vi "Test.vi"() -> ()   [LabVIEW 2014]
doc: "This VI is called when test mode begins, and will automatically be terminated when it ends. You can add manual or automatic tests and invoke them from the dashboard."
uses:
  Robot Global Data.vi
  <vilib>/Rock Robotics/WPI/MotorControl/WPI_MotorControlOpenCANTalonSRX.vi
  <vilib>/Rock Robotics/Network Tables/SD Read String Array.vi
panel:
  in  "Stop":bool
  in  "Motor Power":dbl format="%#_13g"
  in  "Motor":i32(listbox)
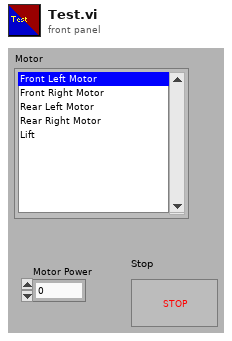
[diagram p1: front panel]
types:
  T1 = typedef "WPI_MotorControlDeviceRef.ctl" = cluster{"DeviceStatus":errorcluster, "Type":T2, "PWM":cluster{"Controller":T3, "PWM Channel":T4, "DeadBand":T5}, "CAN":cluster{"Device Number":u8, "Control Mode":T6, "Semaphore":T7, "Max Vout":dbl, "TalonSRX Control Mode":T8}, "Invert":bool, "TransformRef":T9, "InvTransformRef":T9}
  T2 = typedef "WPI_MotorControlType.ctl" = enum16{"PWM", "CAN", "CANTalonSRX"}
  T3 = typedef "FPGA_TypedefDigitalModule.ctl" = enum16{"Controller 1"}
  T4 = typedef "FPGA_DIOPWMChannel.ctl" = enum8{"PWM 0", "PWM 1", "PWM 2", "PWM 3", "PWM 4", "PWM 5", "PWM 6", "PWM 7", "PWM 8", "PWM 9", "PWM MXP 0", "PWM MXP 1", "PWM MXP 2", "PWM MXP 3", "PWM MXP 4", "PWM MXP 5", "PWM MXP 6", "PWM MXP 7", "PWM MXP 8", "PWM MXP 9", "Invalid"}
  T5 = typedef "WPI_PWMDeadband.ctl" = cluster{"Name":string, "maxPositivePwm":i32, "minPositivePwm":i32, "centerPwm":i32, "maxNegativePwm":i32, "minNegativePwm":i32, "angularRange":u16}
  T6 = typedef "WPI_CANJaguar_ControlMode.ctl" = enum8{"Percent VBus", "Current", "Speed", "Position", "Voltage"}
  T7 = typedef "Semaphore RefNum" = refnum<k1>
  T8 = typedef "WPI_CANTalonSRX_APIControlMode.ctl" = enum8{"Percent VBus", "Speed", "Position", "Slave", "Unchanged / Invalid"}
  T9 = typedef "WPI_PWMTransform_ConPane.ctl" = refnum<vi>
  T10 = typedef "WPI_CANTalonSRX_GlobalStatus.ctl" = cluster{"Applied Throttle":dbl, "Module Enabled":bool, "CAN Error":errorcluster, "Closed Loop Error":dbl, "Forward Limit Switch Closed":bool, "Reverse Limit Switch Closed":bool, "Sensor Position":dbl, "Sensor Velocity":dbl, "Current":dbl, "Sticky Fault - Over Temp":bool, "Sticky Fault - Under Voltage":bool, "Sticky Fault - Forward Limit":bool, "Sticky Fault - Reverse Limit":bool, "Sticky Fault - Forward Soft Limit":bool, "Sticky Fault - Reverse Soft Limit":bool, "Brake is Enabled":bool, "Encoder Position":dbl, "Encoder Velocity":dbl, "Encoder Index Count":dbl, "Encoder A Pin State":bool, "Encoder B Pin State":bool, "Encoder Index Pin State":bool, "Analog In":dbl, "Analog In Velocity":dbl, "Temperature (C)":dbl, "Battery Voltage":dbl}
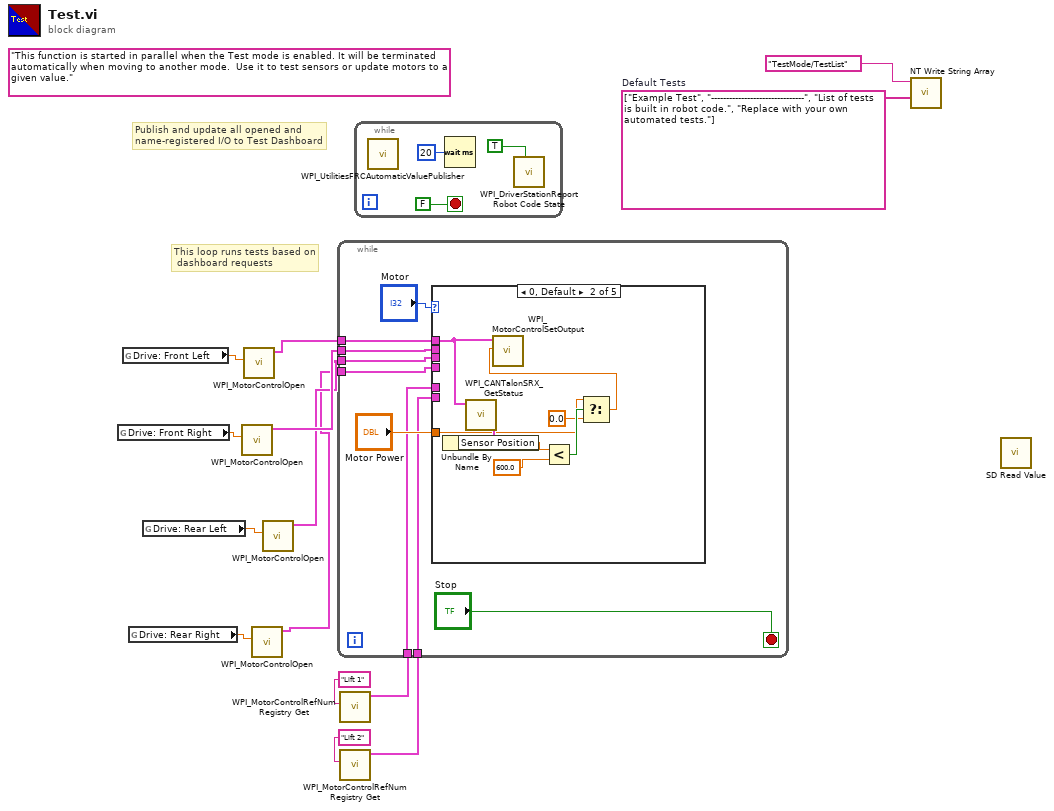
[diagram p0: block diagram]
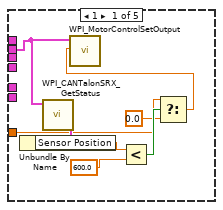
[diagram p2: hidden frame]
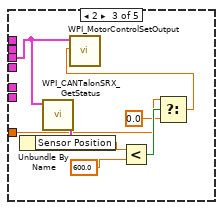
[diagram p3: hidden frame]
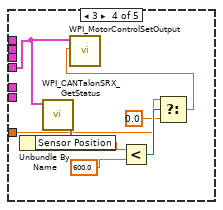
[diagram p4: hidden frame]
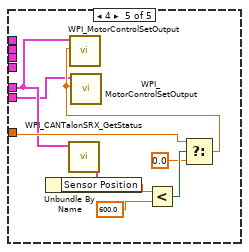
[diagram p5: hidden frame]
diagram:
  w14 = string[] ["Example Test", "-------------------------------", "List of tests is built in robot code.", "Replace with your own automated tests."]  # Default Tests
  (unwired) "This function is started in parallel when the Test mode is enabled. It will be terminated automatically when moving to another mode.  Use it to test sensors or update motors to a given value."
  # "This loop runs tests based on \n dashboard requests"
  # "Publish and update all opened and\nname-registered I/O to Test Dashboard"
  n1 = global read "Robot Global Data.vi" "Drive: Front Right"() -> (w4:dbl)
  n2 = global read "Robot Global Data.vi" "Drive: Front Left"() -> (w8:dbl)
  n3 = global read "Robot Global Data.vi" "Drive: Rear Right"() -> (w6:dbl)
  n4 = global read "Robot Global Data.vi" "Drive: Rear Left"() -> (w7:dbl)
  n5 = call-poly <vilib>:"WPI_MotorControlOpen.vi"("Device Number"=w4) -> ("MotorControlDeviceRef"=w3:T1)  [unwired: 9 in, 1 out]
  n6 = call-poly <vilib>:"WPI_MotorControlOpen.vi"("Device Number"=w8) -> ("MotorControlDeviceRef"=w5:T1)  [unwired: 9 in, 1 out]
  n7 = call-poly <vilib>:"WPI_MotorControlOpen.vi"("Device Number"=w6) -> ("MotorControlDeviceRef"=w1:T1)  [unwired: 9 in, 1 out]
  n8 = call-poly <vilib>:"WPI_MotorControlOpen.vi"("Device Number"=w7) -> ("MotorControlDeviceRef"=w2:T1)  [unwired: 9 in, 1 out]
  n9 = call <vilib>:"WPI_MotorControlRefNum Registry Get.vi"("refnum name"="Lift 1") -> ("MotorControlDevRef"=w10:T1)  [unwired: 9 in, 1 out]
  n10 = call <vilib>:"WPI_MotorControlRefNum Registry Get.vi"("refnum name"="Lift 2") -> ("MotorControlDevRef"=w9:T1)  [unwired: 9 in, 1 out]
  n11 = while {
    tunnel: w5 -> [w23]
    tunnel: w3 -> [w22]
    tunnel: w2 -> [w21]
    tunnel: w1 -> [w20]
    tunnel: w10 -> [w17]
    tunnel: w9 -> [w16]
    stop <- "Stop" stop-if-true
    n12 = case shown="0, Default" "Motor" {
      tunnel: w23 -> [_ w38 _ _ _]
      tunnel: w22 -> [w24 _ _ _ _]
      tunnel: w21 -> [_ _ w40 _ _]
      tunnel: w20 -> [_ _ _ w48 _]
      tunnel: "Motor Power" -> [w27 w34 w43 w51 w60]
      tunnel: w17 -> [_ _ _ _ w58]
      tunnel: w16 -> [_ _ _ _ w56]
      frame 1 {
        n13 = call <vilib>:"WPI_CANTalonSRX_GetStatus.vi"("CAN Talon SRX Ref"=w24) -> ("Talon SRX Status"=w31:T10)  [unwired: 8 in, 2 out]
        n14 = Unbundle By Name(w31) -> ("Sensor Position"=w30:dbl)
        n15 = Less?(x=w30, y=600.0 ("x")) -> (x < y?=w28:bool)
        n16 = Select(t=w27, s=w28, f=0.0) -> (s? t:f=w25:dbl)
        n17 = call <vilib>:"WPI_MotorControlSetOutput.vi"("Output"=w25, "MotorControlDevRef"=w24) -> ()  [unwired: 7 in, 3 out]
      }
      frame 0, Default {
        n18 = call <vilib>:"WPI_CANTalonSRX_GetStatus.vi"("CAN Talon SRX Ref"=w38) -> ("Talon SRX Status"=w39:T10)  [unwired: 8 in, 2 out]
        n19 = Unbundle By Name(w39) -> ("Sensor Position"=w37:dbl)
        n20 = Less?(x=w37, y=600.0 ("x")) -> (x < y?=w35:bool)
        n21 = Select(t=w34, s=w35, f=0.0) -> (s? t:f=w32:dbl)
        n22 = call <vilib>:"WPI_MotorControlSetOutput.vi"("Output"=w32, "MotorControlDevRef"=w38) -> ()  [unwired: 7 in, 3 out]
      }
      frame 2 {
        n23 = call <vilib>:"WPI_CANTalonSRX_GetStatus.vi"("CAN Talon SRX Ref"=w40) -> ("Talon SRX Status"=w47:T10)  [unwired: 8 in, 2 out]
        n24 = Unbundle By Name(w47) -> ("Sensor Position"=w46:dbl)
        n25 = Less?(x=w46, y=600.0 ("x")) -> (x < y?=w44:bool)
        n26 = Select(t=w43, s=w44, f=0.0) -> (s? t:f=w41:dbl)
        n27 = call <vilib>:"WPI_MotorControlSetOutput.vi"("Output"=w41, "MotorControlDevRef"=w40) -> ()  [unwired: 7 in, 3 out]
      }
      frame 3 {
        n28 = call <vilib>:"WPI_CANTalonSRX_GetStatus.vi"("CAN Talon SRX Ref"=w48) -> ("Talon SRX Status"=w55:T10)  [unwired: 8 in, 2 out]
        n29 = Unbundle By Name(w55) -> ("Sensor Position"=w54:dbl)
        n30 = Less?(x=w54, y=600.0 ("x")) -> (x < y?=w52:bool)
        n31 = Select(t=w51, s=w52, f=0.0) -> (s? t:f=w49:dbl)
        n32 = call <vilib>:"WPI_MotorControlSetOutput.vi"("Output"=w49, "MotorControlDevRef"=w48) -> ()  [unwired: 7 in, 3 out]
      }
      frame 4 {
        n33 = call <vilib>:"WPI_CANTalonSRX_GetStatus.vi"("CAN Talon SRX Ref"=w58) -> ("Talon SRX Status"=w64:T10)  [unwired: 8 in, 2 out]
        n34 = Unbundle By Name(w64) -> ("Sensor Position"=w63:dbl)
        n35 = Less?(x=w63, y=600.0 ("x")) -> (x < y?=w61:bool)
        n36 = Select(t=w60, s=w61, f=0.0) -> (s? t:f=w57:dbl)
        n37 = call <vilib>:"WPI_MotorControlSetOutput.vi"("Output"=w57, "MotorControlDevRef"=w58) -> ()  [unwired: 7 in, 3 out]
        n38 = call <vilib>:"WPI_MotorControlSetOutput.vi"("Output"=w57, "MotorControlDevRef"=w56) -> ()  [unwired: 7 in, 3 out]
      }
    }
  }
  n39 = while {
    stop <- FALSE stop-if-true
    n40 = call <vilib>:"WPI_UtilitiesFRCAutomaticValuePublisher.vi"() -> ()  [unwired: 12 in]
    n41 = Wait (ms)(milliseconds to wait=u32 20) -> ()  [unwired: 1 out]
    n42 = call <vilib>:"WPI_DriverStationReport Robot Code State.vi"("Test"=TRUE ("Autonomous")) -> ()  [unwired: 10 in, 1 out]
  }
  n43 = call <vilib>:"NT Write String Array.vi"("String Array"=w14, "Name"="TestMode/TestList") -> ()  [unwired: 9 in, 1 out]
  n44 = call-poly <vilib>:"SD Read Value.vi"() -> ()  [unwired: 10 in, 2 out]
